vi "Cleanup Device.vi"(8 "error in (no error)":errorcluster, 11 "Simulated Waveform in":refnum<class "Simulated Waveform.lvclass">) -> (0 "error out":errorcluster, 3 "Simulated Waveform out":refnum<class "Simulated Waveform.lvclass">)   [LabVIEW 2020, in "Simulated Waveform.lvlib" / "Simulated Waveform.lvclass"]
uses:
  Simulated Waveform.lvclass
  Simulated Waveform.lvclass/Simulated Waveform.ctl
  build/ppl/Signal Generator.lvlibp/Signal Generator/Signal Generator.lvclass
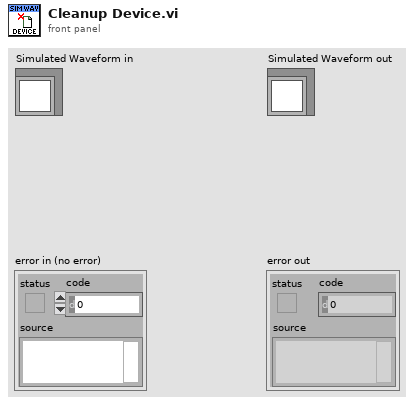
[diagram p1: front panel]
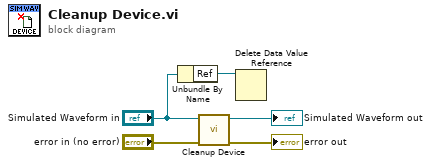
[diagram p0: block diagram]
diagram:
  n1 = Unbundle By Name("Simulated Waveform in") -> ("Ref"=w5:refnum<data-value>)
  n2 = call-parent "Cleanup Device.vi"("error in (no error)"="error in (no error)", "Signal Generator in"="Simulated Waveform in") -> ("error out"=→"error out":errorcluster, "Signal Generator out"=→"Simulated Waveform out":refnum<class "Simulated Waveform.lvclass">)  [unwired: 8 in]
  n3 = Delete Data Value Reference(data value reference=w5) -> ()  [unwired: 1 in, 2 out]
